vi "Check_Aero_Tunnel_on_Server.vi"(0 "Values":dbl[](array[numeric]) format="%.2f", 2 "Ch Names":string[](array[string]), 3 "Current Time":dbl format="%.2f", 4 "Adam Loop Count":i32) -> (6 "Scan comment":string)   [LabVIEW 2011]
uses:
  Controls/In_Range.ctl
panel:
  in  "Tweak time Down":dbl=100.0
  in  "Sec per delta speed down":dbl=1.75
  out "Reset Integral Term":bool
  in  "Tweak time Up":dbl=50.0
  in  "delta t per delta speed":dbl=0.1
  out "Significant speed change?":bool
  out "Valve Dem Pos":dbl
  out "Tweak in working section demanded temp":dbl
  out "Run Aero Chiller PID?":bool
  in  "Delta Speed greater than":dbl=5.0
  in  "Sec per delta speed up":dbl=0.8
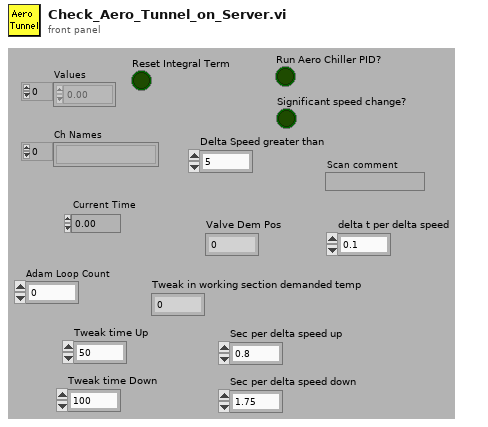
[diagram p1: front panel]
types:
  T1 = typedef "In_Range.ctl" = enum16{"%", "±", "% & ±"}
  T2 = typedef "LVDateTimeRec.ctl" = cluster{"fractional second":dbl, "second":i32, "minute":i32, "hour":i32, "day of month":i32, "month":i32, "year":i32, "day of week":i32, "day of year":i32, "DST":i32}
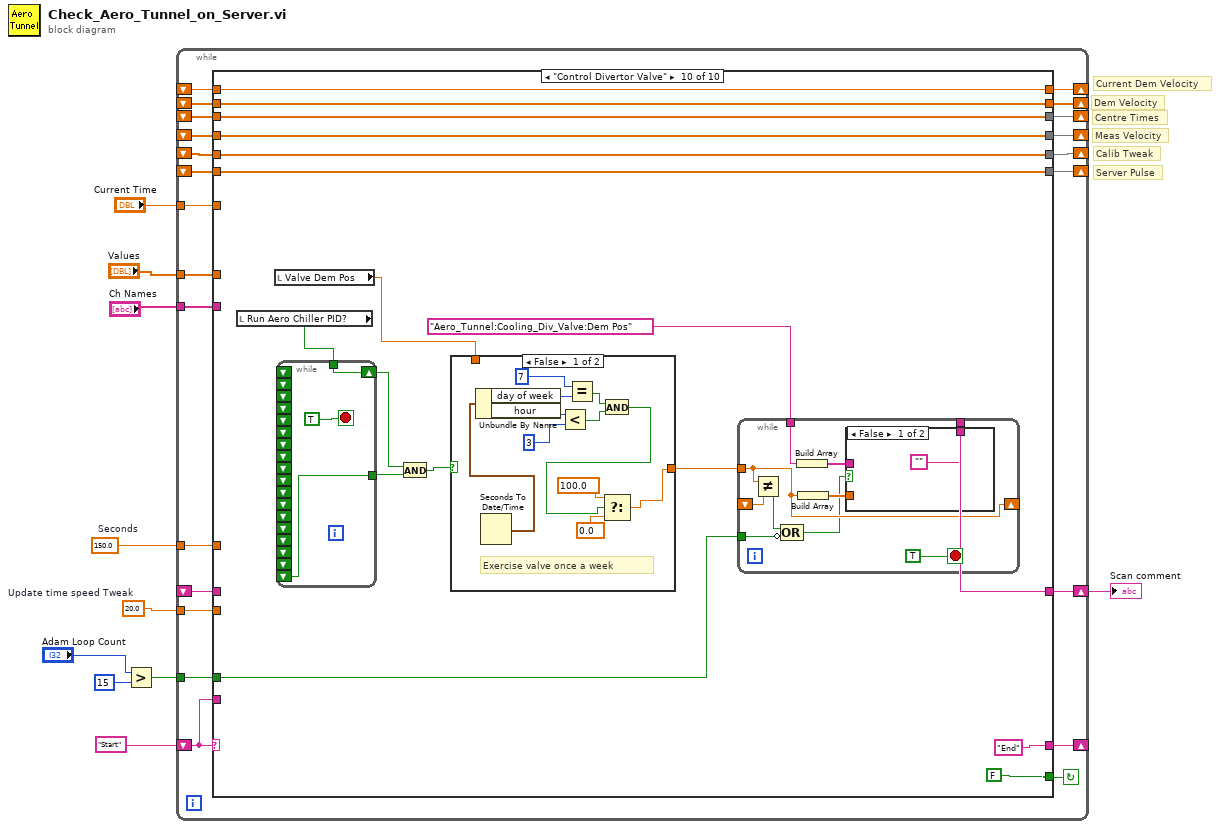
[diagram p0: block diagram]
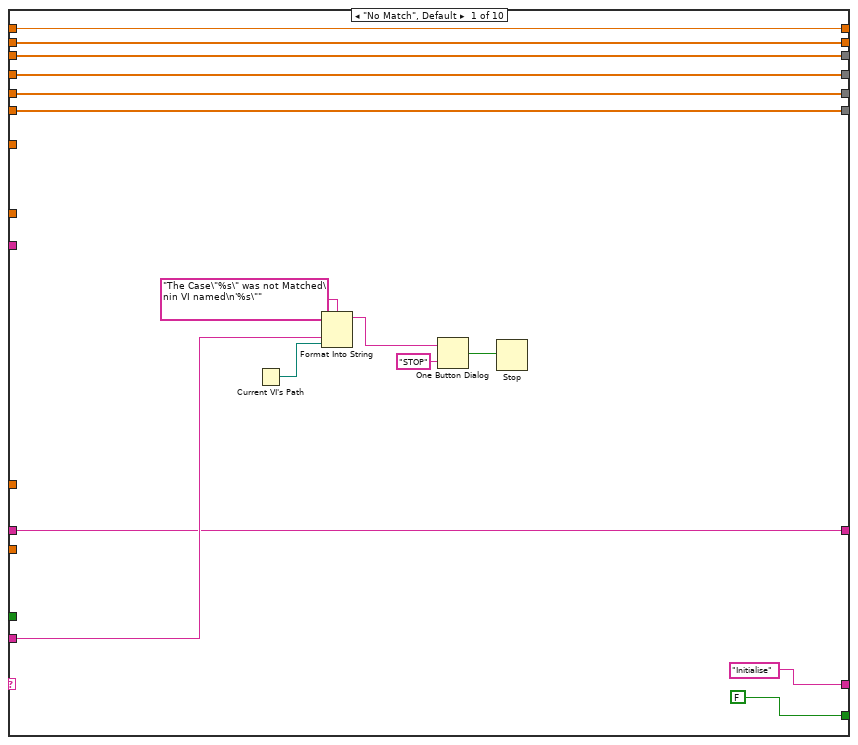
[diagram p2: hidden frame]
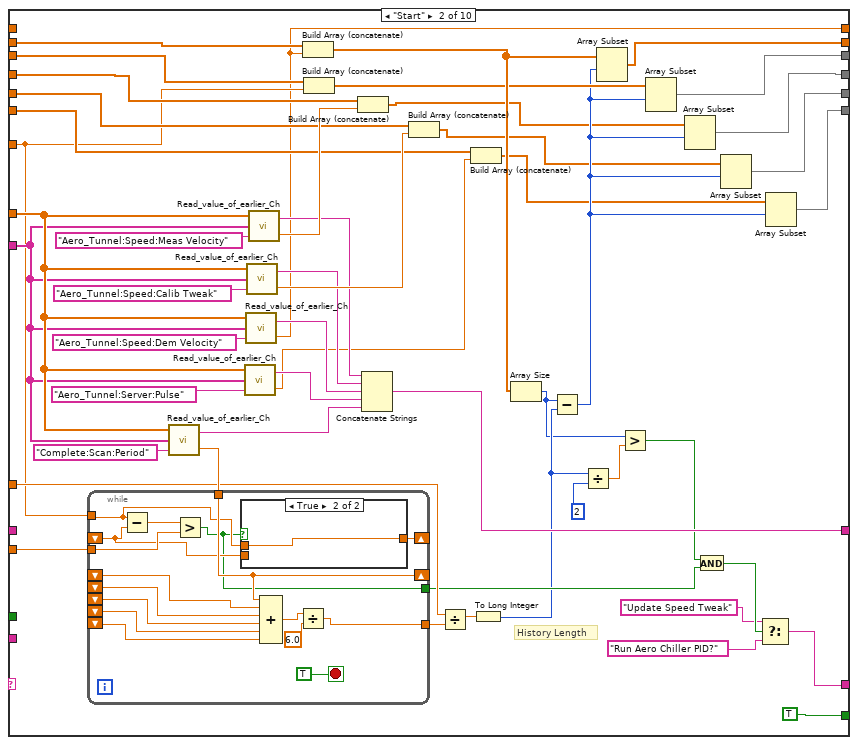
[diagram p3: hidden frame]
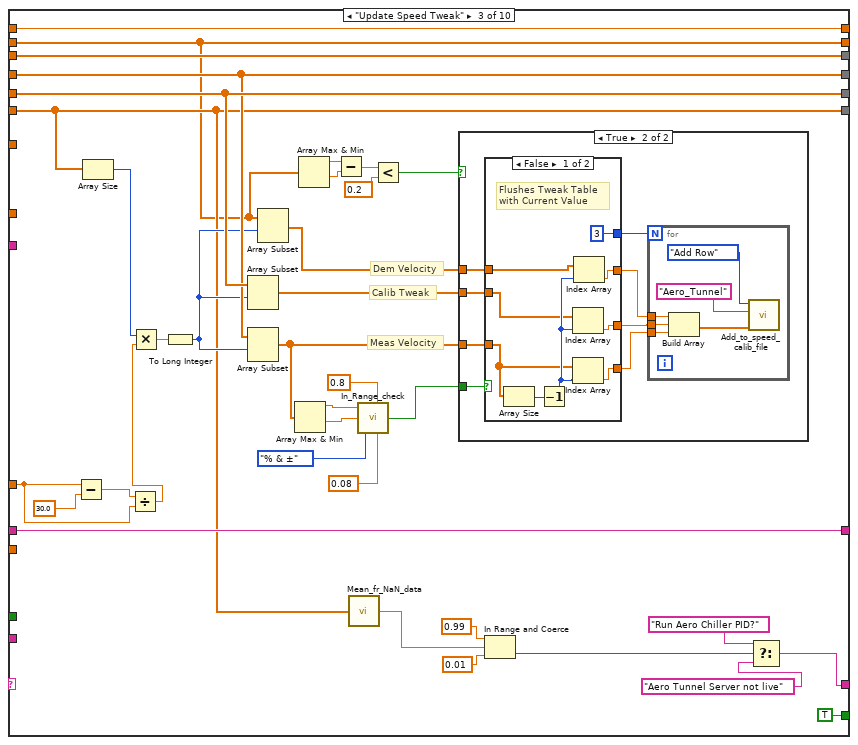
[diagram p5: hidden frame]
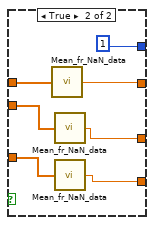
[diagram p7: hidden frame]
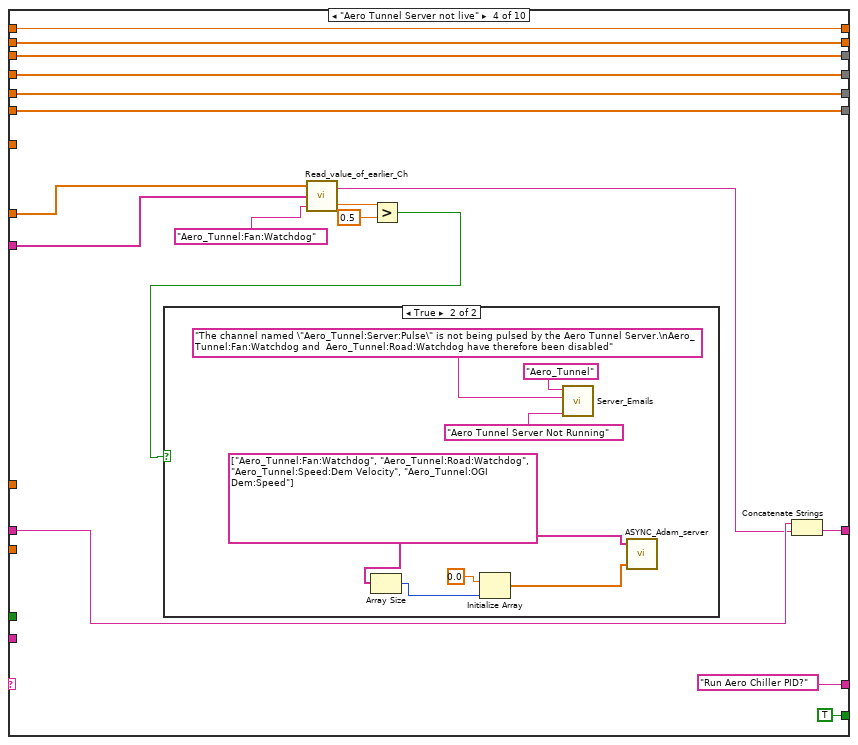
[diagram p8: hidden frame]
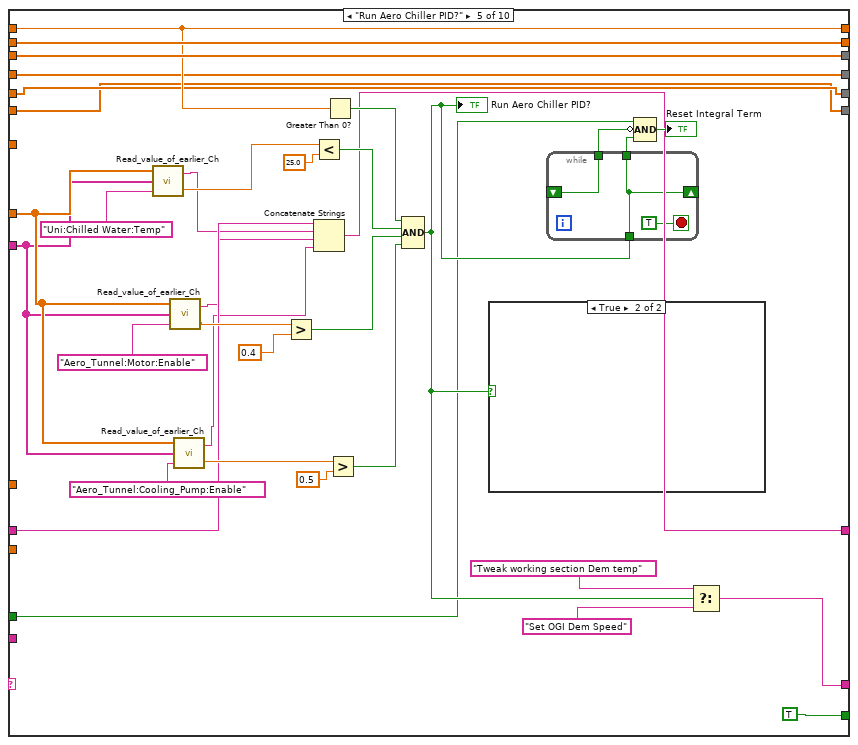
[diagram p10: hidden frame]
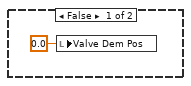
[diagram p11: hidden frame]
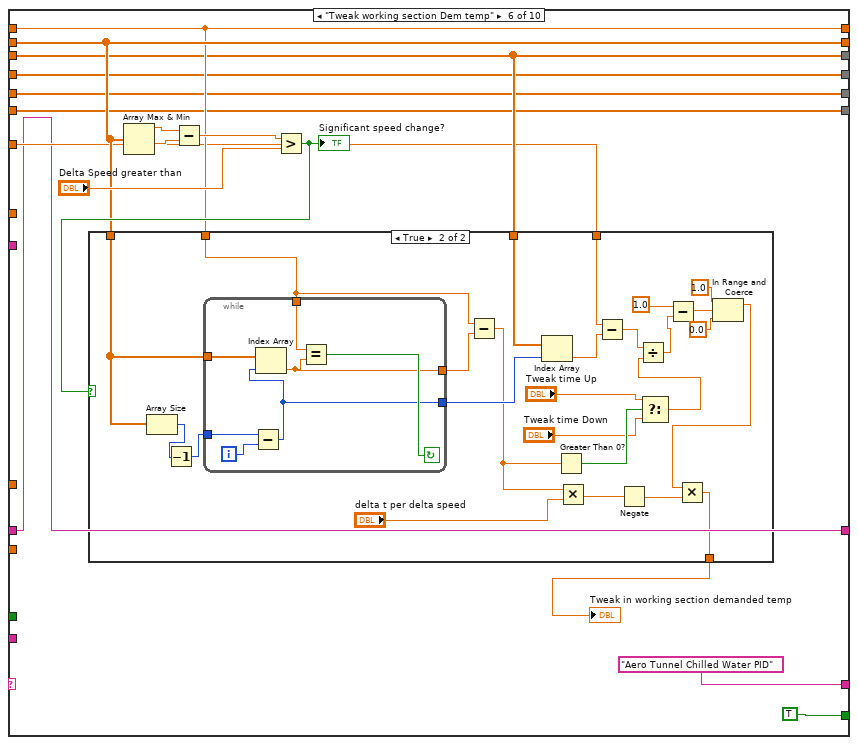
[diagram p12: hidden frame]
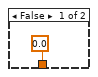
[diagram p13: hidden frame]
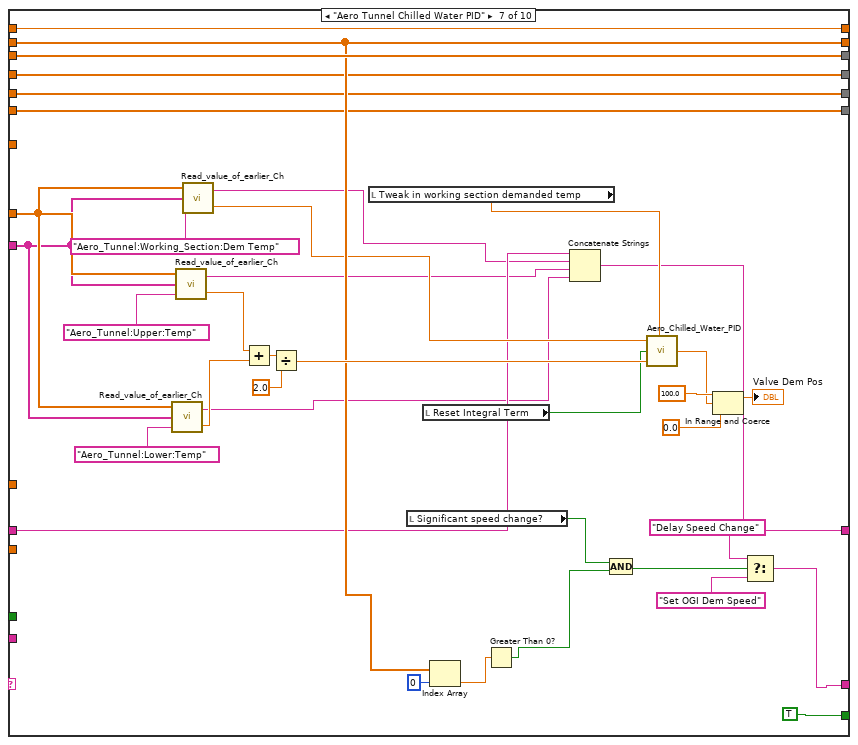
[diagram p14: hidden frame]
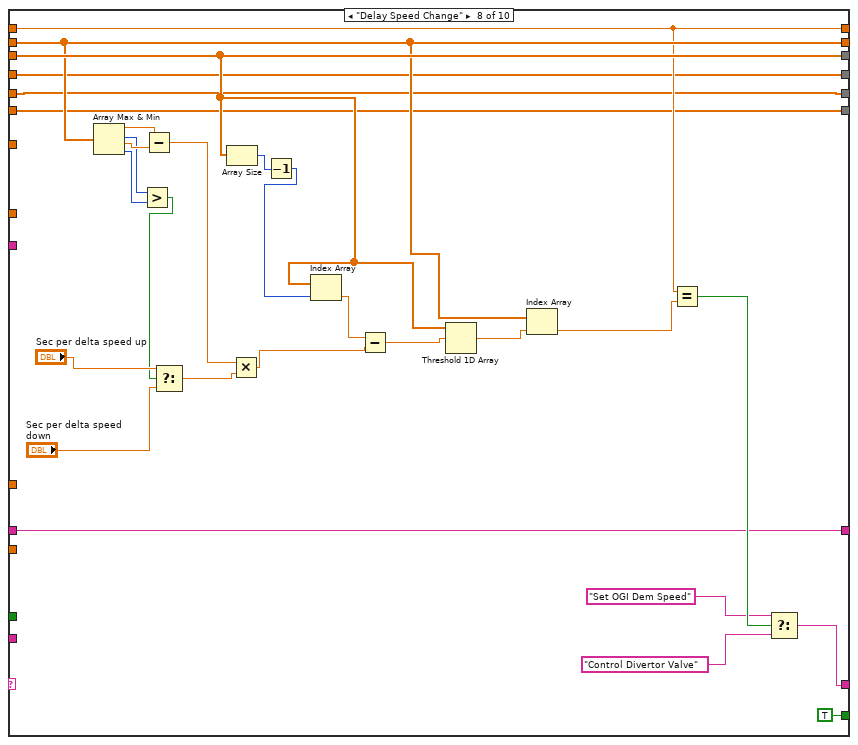
[diagram p15: hidden frame]
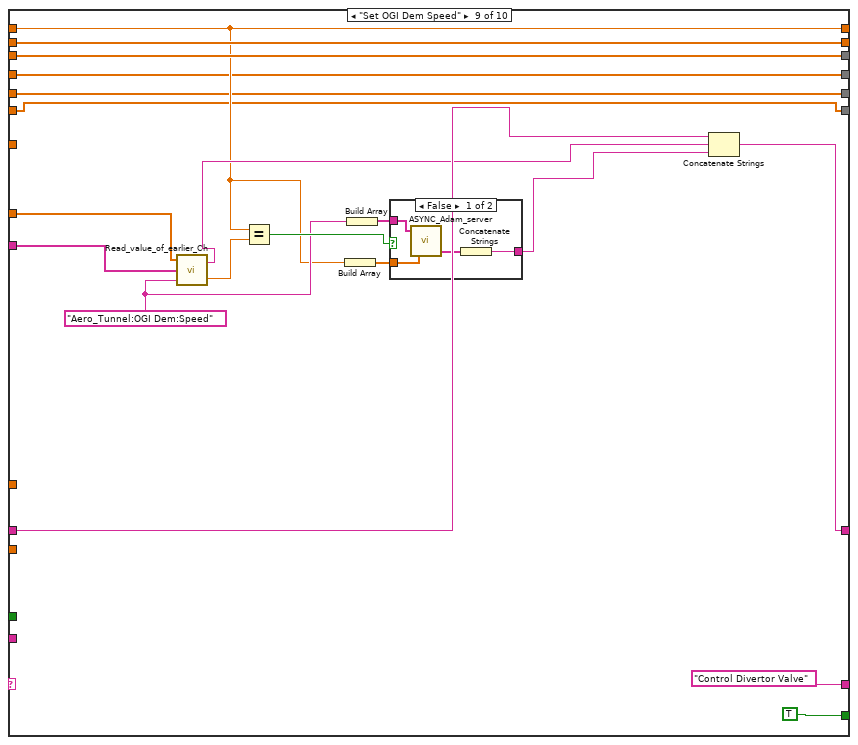
[diagram p16: hidden frame]
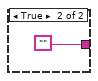
[diagram p17: hidden frame]
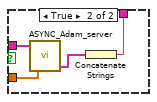
[diagram p19: hidden frame]
diagram:
  w1 = 20.0  # Update time speed Tweak
  w2 = 150.0  # Seconds
  # "Server Pulse"
  # "Calib Tweak"
  # "Meas Velocity"
  # "Dem Velocity"
  # "Centre Times"
  # "Current Dem Velocity"
  n1 = Greater?(x="Adam Loop Count", y=15) -> (0:w4:bool)
  n2 = while {
    shift-left: "Start" -> [w31]
    shift-right: [w32] -> _
    tunnel: "Values" -> [w30]
    tunnel: "Ch Names" -> [w29]
    shift-right: [w28] -> _
    shift-left: _ -> [w27]
    shift-right: [w25] -> _
    shift-left: _ -> [w26]
    shift-right: [w22] -> _
    shift-left: _ -> [w23]
    tunnel: "Current Time" -> [w24]
    tunnel: w4 -> [w21]
    shift-right: [w20] -> w3
    shift-left: _ -> [w19]
    tunnel: w2 -> [w18]
    shift-right: [w17] -> _
    shift-left: _ -> [w16]
    shift-right: [w15] -> _
    shift-left: _ -> [w14]
    shift-right: [w13] -> _
    shift-left: _ -> [w12]
    tunnel: w1 -> [w11]
    stop <- w33 continue-if-true
    n3 = case shown="\"Control Divertor Valve\"" w31 {
      tunnel: [FALSE TRUE TRUE TRUE TRUE TRUE TRUE TRUE TRUE FALSE] -> w33
      tunnel: ["Initialise" w59 w131 "Run Aero Chiller PID?" ("t") w236 "Aero Tunnel Chilled Water PID" w307 w342 "Control Divertor Valve" "End" ("t")] -> w32
      tunnel: w31 -> [w43 _ _ _ _ _ _ _ _ _]
      tunnel: w30 -> [_ w79 _ w189 w222 _ w317 _ w376 _]
      tunnel: w29 -> [_ w78 _ w188 w221 _ w316 _ w375 _]
      tunnel: [w40 w55 w151 w194 w227 w253 w327 w349 w364 w397] -> w28
      tunnel: w27 -> [w40 _ w151 w194 w227 w253 w327 w349 w364 w397]
      tunnel: w26 -> [w39 w93 w123 w195 w235 w254 w311 w350 w369 w399]
      tunnel: [w39 w91 w123 w195 w235 w254 w311 w350 w369 w399] -> w25
      tunnel: w24 -> [_ w65 _ _ _ w251 _ _ _ _]
      tunnel: w23 -> [w38 w89 w150 w196 w234 w252 w329 w351 w368 w398]
      tunnel: [w38 w88 w150 w196 w234 w252 w329 w351 w368 w398] -> w22
      tunnel: w21 -> [_ _ _ _ w216 _ _ _ _ w388]
      tunnel: [w37 w85 w149 w185 w210 w249 w298 w335 w363 w387] -> w20
      tunnel: w19 -> [w37 _ w149 w187 w214 w249 w302 w335 w367 _]
      tunnel: w18 -> [_ w84 w146 _ _ _ _ _ _ _]
      tunnel: [w36 w68 w138 w199 w209 w248 w297 w334 w362 w386] -> w17
      tunnel: w16 -> [w36 w75 w138 w199 w209 w248 w297 w334 w362 w386]
      tunnel: [w35 w67 w139 w198 w208 w247 w296 w333 w361 w385] -> w15
      tunnel: w14 -> [w35 w74 w139 w198 w208 w247 w296 w333 w361 w385]
      tunnel: [w34 w66 w132 w197 w207 w246 w295 w332 w360 w384] -> w13
      tunnel: w12 -> [w34 w73 w132 w197 w207 w246 w295 w332 w360 w384]
      tunnel: w11 -> [_ w64 _ _ _ _ _ _ _ _]
      frame "No Match", Default {
        n4 = Current VI's Path() -> (path=w42:path)
        n5 = Format Into String(format string="The Case\"%s\" was not Matched\nin VI named\n'%s\"" ("Format String"), w43, w42) -> (resulting string=w46:string)  [unwired: 2 in, 1 out]
        n6 = One Button Dialog(message=w46, button name ("OK")="STOP") -> (true=w44:bool)
        n7 = Stop(stop? (T)=w44) -> ()
      }
      frame "Start" {
        # "History Length"
        n8 = call "Read_value_of_earlier_Ch.vi"("Desired Ch to Read"="Complete:Scan:Period", "Ch names"=w78, "Present scan array"=w79) -> ("Value"=w95:dbl, "Scan comment"=w86:string)  [unwired: 1 in]
        n9 = while {
          shift-right: [w114] -> _
          shift-left: _ -> [w113]
          tunnel: w95 -> [w114]
          shift-left: _ -> [w112]
          shift-left: _ -> [w111]
          shift-left: _ -> [w110]
          shift-left: _ -> [w109]
          tunnel: [w105] -> w94
          tunnel: w65 -> [w101]
          shift-right: [w102] -> _
          shift-left: _ -> [w100]
          tunnel: w64 -> [w103]
          tunnel: [w99] -> w63
          stop <- TRUE stop-if-true
          n10 = Subtract(x=w101, y=w100) -> (x-y=w104:dbl)
          n11 = Greater?(x=w104, y=w103) -> (0:w99:bool)
          n12 = case shown="True" w99 {
            tunnel: [w115 w116] -> w102
            tunnel: w101 -> [_ w116]
            tunnel: w100 -> [w115 _]
            frame False {
            }
            frame True {
            }
          }
          n13 = Compound Arithmetic op=ADD(w114, w113, w112, w111, w110, w109) -> (w107:dbl)
          n14 = Divide(x=w107, y=6.0) -> (x/y=w105:dbl)
        }
        n15 = call "Read_value_of_earlier_Ch.vi"("Desired Ch to Read"="Aero_Tunnel:Server:Pulse", "Ch names"=w78, "Present scan array"=w79) -> ("Value"=w54:dbl, "Scan comment"=w87:string)  [unwired: 1 in]
        n16 = call "Read_value_of_earlier_Ch.vi"("Desired Ch to Read"="Aero_Tunnel:Speed:Dem Velocity", "Ch names"=w78, "Present scan array"=w79) -> ("Value"=w55:dbl, "Scan comment"=w56:string)  [unwired: 1 in]
        n17 = call "Read_value_of_earlier_Ch.vi"("Desired Ch to Read"="Aero_Tunnel:Speed:Calib Tweak", "Ch names"=w78, "Present scan array"=w79) -> ("Value"=w76:dbl, "Scan comment"=w57:string)  [unwired: 1 in]
        n18 = call "Read_value_of_earlier_Ch.vi"("Desired Ch to Read"="Aero_Tunnel:Speed:Meas Velocity", "Ch names"=w78, "Present scan array"=w79) -> ("Value"=w77:dbl, "Scan comment"=w58:string)  [unwired: 1 in]
        n19 = Build Array (concatenate)(w93, w55) -> (w90:dbl[])
        n20 = Build Array (concatenate)(w89, w65) -> (w80:dbl[])
        n21 = Build Array (concatenate)(w75, w77) -> (w71:dbl[])
        n22 = Concatenate Strings(w58, w57, w56, w87, w86) -> (w85:string)
        n23 = Build Array (concatenate)(w74, w76) -> (w70:dbl[])
        n24 = Divide(x=w84, y=w94) -> (x/y=w92:dbl)
        n25 = Build Array (concatenate)(w73, w54) -> (w69:dbl[])
        n26 = To Long Integer(number=w92) -> (32bit integer=w52:i32)
        n27 = Array Size(array=w90) -> (size(s)=w51:i32)
        n28 = Subtract(x=w51, y=w52) -> (x-y=w72:i32)
        n29 = Divide(x=w52, y=2) -> (x/y=w50:dbl)
        n30 = Array Subset(array=w90, index=w72) -> (w91:dbl[])  [unwired: 1 in]
        n31 = Greater?(x=w51, y=w50) -> (0:w49:bool)
        n32 = Array Subset(array=w80, index=w72) -> (w88:dbl[])  [unwired: 1 in]
        n33 = Array Subset(array=w71, index=w72) -> (w68:dbl[])  [unwired: 1 in]
        n34 = And(x=w49, y=w63) -> (x .and. y?=w62:bool)
        n35 = Array Subset(array=w70, index=w72) -> (w67:dbl[])  [unwired: 1 in]
        n36 = Select(t="Update Speed Tweak", s=w62, f="Run Aero Chiller PID?" ("t")) -> (s? t:f=w59:string)
        n37 = Array Subset(array=w69, index=w72) -> (w66:dbl[])  [unwired: 1 in]
      }
      frame "Update Speed Tweak" {
        # "Meas Velocity"
        # "Calib Tweak"
        # "Dem Velocity"
        n38 = Subtract(x=w146, y=30.0) -> (x-y=w147:dbl)
        n39 = Array Size(array=w132) -> (size(s)=w124:i32)
        n40 = Divide(x=w147, y=w146) -> (x/y=w145:dbl)
        n41 = Multiply(x=w124, y=w145) -> (x*y=w144:dbl)
        n42 = To Long Integer(number=w144) -> (32bit integer=w134:i32)
        n43 = Array Subset(array=w139, index=w134) -> (w126:dbl[])  [unwired: 1 in]
        n44 = Array Subset(array=w138, index=w134) -> (w125:dbl[])  [unwired: 1 in]
        n45 = Array Subset(array=w123, index=w134) -> (w127:dbl[])  [unwired: 1 in]
        n46 = Array Max & Min(array=w125) -> (max value=w122:dbl, min value=w121:dbl)  [unwired: 2 out]
        n47 = Array Max & Min(array=w123) -> (max value=w143:dbl, min value=w142:dbl)  [unwired: 2 out]
        n48 = Subtract(x=w143, y=w142) -> (x-y=w141:dbl)
        n49 = call "Mean_fr_NaN_data.vi"("Data"=w132) -> ("Mean value"=w133:dbl)
        n50 = call "In_Range_check.vi"("±"=0.08, "%"=0.8, "Mode"=In_Range."% & ±", "Value"=w121, "Setpoint"=w122) -> ("In Range"=w117:bool)  [unwired: 2 out]
        n51 = Less?(x=w141, y=0.2) -> (x < y?=w137:bool)
        n52 = case shown="True" w137 {
          tunnel: w127 -> [_ w160]
          tunnel: w126 -> [_ w159]
          tunnel: w125 -> [_ w158]
          tunnel: w117 -> [_ w154]
          frame False {
          }
          frame True {
            n53 = case shown="False" w154 {
              tunnel: w160 -> [w173 w182]
              tunnel: w159 -> [w172 w181]
              tunnel: w158 -> [w171 w180]
              tunnel: [w170 w179] -> w157
              tunnel: [w169 w178] -> w156
              tunnel: [w168 w177] -> w155
              tunnel: [3 1] -> w153
              frame False {
                # "Flushes Tweak Table\nwith Current Value"
                n54 = Array Size(array=w171) -> (size(s)=w175:i32)
                n55 = Decrement(x=w175) -> (x-1=w174:i32)
                n56 = Index Array(array=w172, index=w174) -> (element=w169:dbl)
                n57 = Index Array(array=w171, index=w174) -> (element=w170:dbl)
                n58 = Index Array(array=w173, index=w174) -> (element=w168:dbl)
              }
              frame True {
                n59 = call "Mean_fr_NaN_data.vi"("Data"=w182) -> ("Mean value"=w177:dbl)
                n60 = call "Mean_fr_NaN_data.vi"("Data"=w181) -> ("Mean value"=w178:dbl)
                n61 = call "Mean_fr_NaN_data.vi"("Data"=w180) -> ("Mean value"=w179:dbl)
              }
            }
            n62 = for {
              N: w153 -> [_]
              tunnel: w157 -> [w163]
              tunnel: w156 -> [w162]
              tunnel: w155 -> [w161]
              n63 = Build Array(w161, w162, w163) -> (w164:dbl[])
              n64 = call "Add_to_speed_calib_file.vi"("New Row"=w164, "Rig Name"="Aero_Tunnel" ("y"), "Mode"=enum16{"Add Row", "Get Error Value"}."Add Row") -> ()  [unwired: 3 in, 2 out]
            }
          }
        }
        n65 = In Range and Coerce(upper limit=0.99, x=w133, lower limit=0.01) -> (In Range?=w130:bool)  [unwired: 1 out]
        n66 = Select(t="Run Aero Chiller PID?", s=w130, f="Aero Tunnel Server not live" ("t")) -> (s? t:f=w131:string)
      }
      frame "Aero Tunnel Server not live" {
        n67 = call "Read_value_of_earlier_Ch.vi"("Desired Ch to Read"="Aero_Tunnel:Fan:Watchdog", "Ch names"=w188, "Present scan array"=w189) -> ("Value"=w191:dbl, "Scan comment"=w186:string)  [unwired: 1 in]
        n68 = Greater?(x=w191, y=0.5) -> (0:w193:bool)
        n69 = case shown="True" w193 {
          frame False {
          }
          frame True {
            w201 = string[] ["Aero_Tunnel:Fan:Watchdog", "Aero_Tunnel:Road:Watchdog", "Aero_Tunnel:Speed:Dem Velocity", "Aero_Tunnel:OGI Dem:Speed"] ("Channel Names")
            n70 = Array Size(array=w201) -> (size(s)=w202:i32)
            n71 = Initialize Array(0.0, w202) -> (w200:dbl[])
            n72 = call "Server_Emails.vi"("Client Name Contains"="Aero_Tunnel", "Message"="The channel named \"Aero_Tunnel:Server:Pulse\" is not being pulsed by the Aero Tunnel Server.\nAero_Tunnel:Fan:Watchdog and  Aero_Tunnel:Road:Watchdog have therefore been disabled", "Subject"="Aero Tunnel Server Not Running" ("Error Type")) -> ()  [unwired: 2 in, 3 out]
            n73 = call "ASYNC_Adam_server.vi"("Values"=w200, "Channel Names"=w201) -> ()  [unwired: 1 in, 3 out]
          }
        }
        n74 = Concatenate Strings(w187, w186) -> (w185:string)
      }
      frame "Run Aero Chiller PID?" {
        n75 = call "Read_value_of_earlier_Ch.vi"("Desired Ch to Read"="Uni:Chilled Water:Temp", "Ch names"=w221, "Present scan array"=w222) -> ("Value"=w239:dbl, "Scan comment"=w213:string)  [unwired: 1 in]
        n76 = call "Read_value_of_earlier_Ch.vi"("Desired Ch to Read"="Aero_Tunnel:Motor:Enable", "Ch names"=w221, "Present scan array"=w222) -> ("Value"=w230:dbl, "Scan comment"=w212:string)  [unwired: 1 in]
        n77 = call "Read_value_of_earlier_Ch.vi"("Desired Ch to Read"="Aero_Tunnel:Cooling_Pump:Enable", "Ch names"=w221, "Present scan array"=w222) -> ("Value"=w224:dbl, "Scan comment"=w211:string)  [unwired: 1 in]
        n78 = Greater?(x=w230, y=0.4) -> (0:w228:bool)
        n79 = Less?(x=w239, y=25.0) -> (x < y?=w229:bool)
        n80 = Concatenate Strings(w214, w213, w212, w211) -> (w210:string)
        n81 = Greater Than 0?(x=w227) -> (x > 0?=w226:bool)
        n82 = Greater?(x=w224, y=0.5) -> (0:w220:bool)
        n83 = Compound Arithmetic op=AND(w226, w229, w228, w220) -> (w219:bool)
        "Run Aero Chiller PID?" <- w219
        n84 = case shown="True" w219 {
          frame False {
            n85 = local write "Valve Dem Pos"(0.0 ("Valve Dem Pos")) -> ()
          }
          frame True {
          }
        }
        n86 = while {
          shift-right: [w243] -> _
          shift-left: _ -> [w244]
          tunnel: w219 -> [w243]
          tunnel: [w244] -> w218
          tunnel: [w243] -> w217
          stop <- TRUE stop-if-true
        }
        n87 = Compound Arithmetic op=AND(w216, invert w218, w217) -> (→"Reset Integral Term":bool)
        n88 = Select(t="Tweak working section Dem temp", s=w219, f="Set OGI Dem Speed") -> (s? t:f=w236:string)
      }
      frame "Tweak working section Dem temp" {
        n89 = Array Max & Min(array=w254) -> (max value=w258:dbl, min value=w259:dbl)  [unwired: 2 out]
        n90 = Subtract(x=w258, y=w259) -> (x-y=w257:dbl)
        n91 = Greater?(x=w257, y="Delta Speed greater than") -> (0:w255:bool)
        "Significant speed change?" <- w255
        n92 = case shown="True" w255 {
          tunnel: w254 -> [_ w286]
          tunnel: w253 -> [_ w280]
          tunnel: w252 -> [_ w283]
          tunnel: w251 -> [_ w282]
          tunnel: [0.0 w270] -> w250
          frame False {
          }
          frame True {
            n93 = Array Size(array=w286) -> (size(s)=w285:i32)
            n94 = Decrement(x=w285) -> (x-1=w287:i32)
            n95 = while {
              tunnel: w287 -> [w293]
              tunnel: w286 -> [w292]
              tunnel: w280 -> [w291]
              tunnel: [w289] -> w284
              tunnel: [w288] -> w279
              i -> [w294]
              stop <- w290 continue-if-true
              n96 = Subtract(x=w293, y=w294) -> (x-y=w289:i32)
              n97 = Index Array(array=w292, index=w289) -> (element=w288:dbl)
              n98 = Equal?(x=w291, y=w288) -> (x = y?=w290:bool)
            }
            n99 = Subtract(x=w280, y=w279) -> (x-y=w267:dbl)
            n100 = Index Array(array=w283, index=w284) -> (element=w281:dbl)
            n101 = Greater Than 0?(x=w267) -> (x > 0?=w266:bool)
            n102 = Multiply(x=w267, y="delta t per delta speed") -> (x*y=w269:dbl)
            n103 = Subtract(x=w282, y=w281) -> (x-y=w276:dbl)
            n104 = Negate(x=w269) -> (-x=w268:dbl)
            n105 = Select(t="Tweak time Up", s=w266, f="Tweak time Down") -> (s? t:f=w263:dbl)
            n106 = Divide(x=w276, y=w263) -> (x/y=w275:dbl)
            n107 = Subtract(x=1.0, y=w275) -> (x-y=w274:dbl)
            n108 = In Range and Coerce(upper limit=1.0, x=w274, lower limit=0.0) -> (coerced(x)=w271:dbl)  [unwired: 1 out]
            n109 = Multiply(x=w271, y=w268) -> (x*y=w270:dbl)
          }
        }
        "Tweak in working section demanded temp" <- w250
      }
      frame "Aero Tunnel Chilled Water PID" {
        n110 = call "Read_value_of_earlier_Ch.vi"("Desired Ch to Read"="Aero_Tunnel:Lower:Temp", "Ch names"=w316, "Present scan array"=w317) -> ("Value"=w320:dbl, "Scan comment"=w299:string)  [unwired: 1 in]
        n111 = call "Read_value_of_earlier_Ch.vi"("Desired Ch to Read"="Aero_Tunnel:Upper:Temp", "Ch names"=w316, "Present scan array"=w317) -> ("Value"=w321:dbl, "Scan comment"=w300:string)  [unwired: 1 in]
        n112 = call "Read_value_of_earlier_Ch.vi"("Desired Ch to Read"="Aero_Tunnel:Working_Section:Dem Temp", "Ch names"=w316, "Present scan array"=w317) -> ("Value"=w303:dbl, "Scan comment"=w301:string)  [unwired: 1 in]
        n113 = Add(x=w321, y=w320) -> (x+y=w322:dbl)
        n114 = Divide(x=w322, y=2.0) -> (x/y=w319:dbl)
        n115 = local read "Tweak in working section demanded temp"() -> (w304:dbl)
        n116 = local read "Significant speed change?"() -> (w306:bool)
        n117 = local read "Reset Integral Term"() -> (w305:bool)
        n118 = Index Array(array=w311, index=0) -> (element=w313:dbl)
        n119 = Greater Than 0?(x=w313) -> (x > 0?=w312:bool)
        n120 = Concatenate Strings(w302, w301, w300, w299) -> (w298:string)
        n121 = Compound Arithmetic op=AND(w306, w312) -> (w308:bool)
        n122 = call "Aero_Chilled_Water_PID.vi"("Tweak in working section demanded temp"=w304, "Present Value"=w319, "Reset PID"=w305, "Setpoint"=w303) -> ("Dem Output"=w324:dbl)
        n123 = In Range and Coerce(upper limit=100.0, x=w324, lower limit=0.0) -> (coerced(x)=→"Valve Dem Pos":dbl)  [unwired: 1 out]
        n124 = Select(t="Delay Speed Change", s=w308, f="Set OGI Dem Speed") -> (s? t:f=w307:string)
      }
      frame "Delay Speed Change" {
        n125 = Array Max & Min(array=w350) -> (max value=w358:dbl, max index (indices)=w341:i32, min value=w359:dbl, min index (indices)=w340:i32)
        n126 = Greater?(x=w341, y=w340) -> (0:w337:bool)
        n127 = Subtract(x=w358, y=w359) -> (x-y=w348:dbl)
        n128 = Select(t="Sec per delta speed up", s=w337, f="Sec per delta speed down") -> (s? t:f=w336:dbl)
        n129 = Array Size(array=w351) -> (size(s)=w353:i32)
        n130 = Multiply(x=w348, y=w336) -> (x*y=w347:dbl)
        n131 = Decrement(x=w353) -> (x-1=w352:i32)
        n132 = Index Array(array=w351, index=w352) -> (element=w354:dbl)
        n133 = Subtract(x=w354, y=w347) -> (x-y=w355:dbl)
        n134 = Threshold 1D Array(2:w355, 3:w351) -> (0:w356:dbl)  [unwired: 1 out]
        n135 = Index Array(array=w350, index=w356) -> (element=w357:dbl)
        n136 = Equal?(x=w349, y=w357) -> (x = y?=w345:bool)
        n137 = Select(t="Set OGI Dem Speed", s=w345, f="Control Divertor Valve") -> (s? t:f=w342:string)
      }
      frame "Set OGI Dem Speed" {
        w372 = "Aero_Tunnel:OGI Dem:Speed"
        n138 = call "Read_value_of_earlier_Ch.vi"("Desired Ch to Read"=w372, "Ch names"=w375, "Present scan array"=w376) -> ("Value"=w374:dbl, "Scan comment"=w366:string)  [unwired: 1 in]
        n139 = Equal?(x=w364, y=w374) -> (x = y?=w373:bool)
        n140 = Build Array(w364) -> (w370:dbl[])
        n141 = Build Array(w372) -> (w371:string[])
        n142 = case shown="False" w373 {
          tunnel: w370 -> [w382 _]
          tunnel: w371 -> [w381 _]
          tunnel: [w379 ""] -> w365
          frame False {
            n143 = call "ASYNC_Adam_server.vi"("Values"=w382, "Channel Names"=w381) -> ("Scan Comments"=w380:string[])  [unwired: 1 in, 2 out]
            n144 = Concatenate Strings(w380) -> (w379:string)
          }
          frame True {
          }
        }
        n145 = Concatenate Strings(w367, w366, w365) -> (w363:string)
      }
      frame "Control Divertor Valve" {
        n146 = local read "Run Aero Chiller PID?"() -> (w390:bool)
        n147 = local read "Valve Dem Pos"() -> (w389:dbl)
        n148 = while {
          shift-right: [w430] -> w391
          shift-left: _ -> [_]
          tunnel: w390 -> [w430]
          shift-left: _ -> [_]
          shift-left: _ -> [_]
          shift-left: _ -> [_]
          shift-left: _ -> [_]
          shift-left: _ -> [_]
          shift-left: _ -> [_]
          shift-left: _ -> [_]
          shift-left: _ -> [_]
          shift-left: _ -> [_]
          shift-left: _ -> [_]
          shift-left: _ -> [_]
          shift-left: _ -> [_]
          shift-left: _ -> [_]
          shift-left: _ -> [_]
          shift-left: _ -> [_]
          shift-left: _ -> [_]
          shift-left: _ -> [w429]
          tunnel: [w429] -> w393
          stop <- TRUE stop-if-true
        }
        n149 = And(x=w391, y=w393) -> (x .and. y?=w394:bool)
        n150 = case shown="False" w394 {
          tunnel: [w402 w412] -> w395
          tunnel: w389 -> [_ w412]
          frame False {
            # "Exercise valve once a week"
            n151 = Seconds To Date/Time() -> (date time rec=w403:T2)  [unwired: 2 out]
            n152 = Unbundle By Name(w403) -> ("day of week"=w408:i32, "hour"=w406:i32)
            n153 = Less?(x=w406, y=3) -> (x < y?=w411:bool)
            n154 = Equal?(x=7, y=w408) -> (x = y?=w410:bool)
            n155 = And(x=w410, y=w411) -> (x .and. y?=w401:bool)
            n156 = Select(t=100.0, s=w401, f=0.0) -> (s? t:f=w402:dbl)
          }
          frame True {
          }
        }
        n157 = while {
          shift-right: [w418] -> _
          shift-left: _ -> [w419]
          tunnel: w395 -> [w418]
          tunnel: "Aero_Tunnel:Cooling_Div_Valve:Dem Pos" -> [w420]
          tunnel: w388 -> [w415]
          tunnel: [w413] -> w387
          stop <- TRUE stop-if-true
          n158 = Not Equal?(x=w418, y=w419) -> (x != y?=w416:bool)
          n159 = Compound Arithmetic op=OR(w416, invert w415) -> (w414:bool)
          n160 = Build Array(w420) -> (w421:string[])
          n161 = Build Array(w418) -> (w422:dbl[])
          n162 = case shown="False" w414 {
            tunnel: w422 -> [_ w427]
            tunnel: w421 -> [_ w426]
            tunnel: ["" w424] -> w413
            frame False {
            }
            frame True {
              n163 = call "ASYNC_Adam_server.vi"("Values"=w427, "Channel Names"=w426) -> ("Scan Comments"=w425:string[])  [unwired: 1 in, 2 out]
              n164 = Concatenate Strings(w425) -> (w424:string)
            }
          }
        }
      }
    }
  }
  "Scan comment" <- w3
